vi "PH_Beckhoff_Application.ProcPeriodic.vi"(0 "i ref in":refnum<vi>, 3 "ms timeout (10000)":i32=10000, 5 "error in (no error)":errorcluster) -> (14 "i ref out":refnum<vi>, 17 "timed out":bool, 19 "error out":errorcluster)   [LabVIEW 2014, in "PH_Beckhoff_Application.lvlib"]
doc: "This method serves to periodically do things like reading values from the HW. Methods that should be executed periodically should be called from THIS methode. Add code here."
uses:
  PH_Beckhoff_Application.lvlib
  PH_Beckhoff/PH_Beckhoff.lvlib
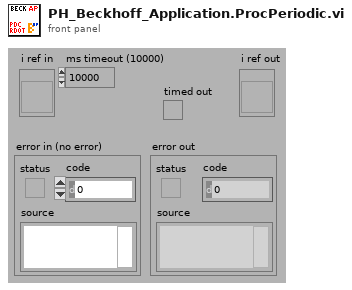
[diagram p1: front panel]
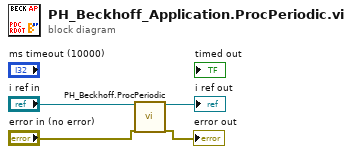
[diagram p0: block diagram]
diagram:
  n1 = call "PH_Beckhoff.ProcPeriodic.vi"("i ref in"="i ref in", "error in (no error)"="error in (no error)") -> ("i ref out"=→"i ref out":refnum<vi>, "error out"=→"error out":errorcluster)  [unwired: 15 in, 1 out]
